vi "write_to_database.vi"(0 "heat_board_control in":refnum<class "heat_board_control.lvclass">, 5 "best setpoint":dbl, 7 "best manual laser":dbl, 11 "error in (no error)":errorcluster, 12 "database connection":path) -> (4 "heat_board_control out":refnum<class "heat_board_control.lvclass">, 15 "error out":errorcluster)   [LabVIEW 2015]
uses:
  heat_board_control.lvclass
  <vilib>/addons/database/Connection.llb/DB Tools Open Connec (Path).vi
  <vilib>/addons/database/NI_Database_API.lvlib
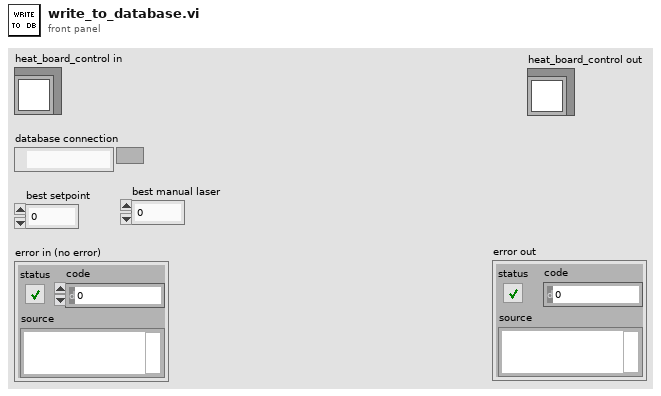
[diagram p1: front panel]
types:
  T1 = typedef "NI_Database_API.lvlib/Conn ObjectReference.ctl" = refnum<k1>
  T2 = cluster{"Rounded Number":dbl, "physical channel":refnum<k21>}
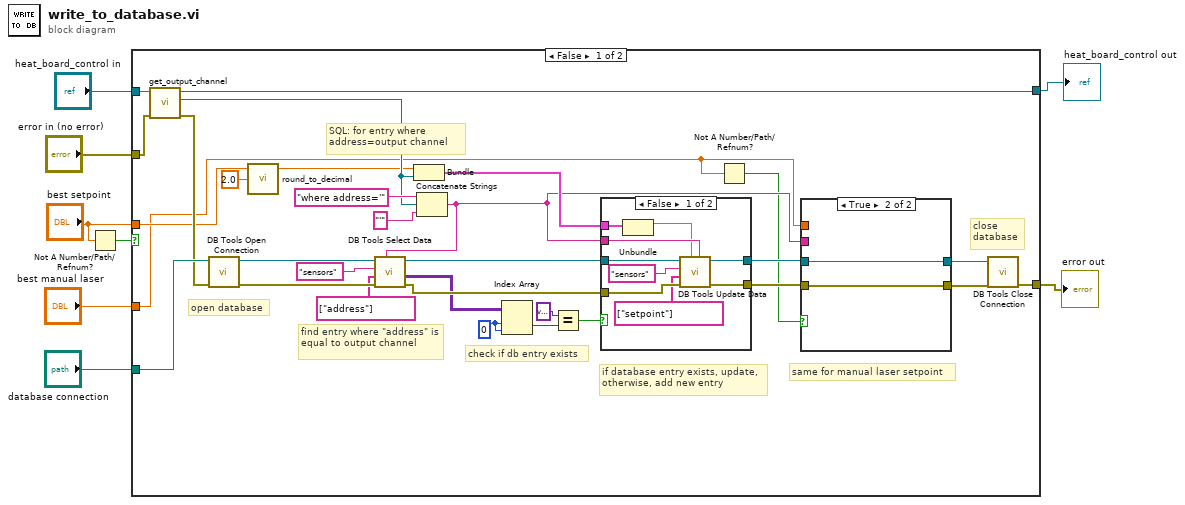
[diagram p0: block diagram]
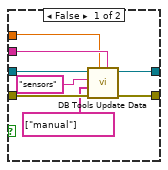
[diagram p2: hidden frame]
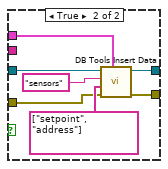
[diagram p3: hidden frame]
diagram:
  n1 = Not A Number/Path/Refnum?(number/path/refnum="best setpoint") -> (NaN/Path/Refnum?=w2:bool)
  n2 = case shown="False" w2 {
    tunnel: "error in (no error)" -> [w39 w66]
    tunnel: [w38 w66] -> w7
    tunnel: "heat_board_control in" -> [w37 w67]
    tunnel: "best setpoint" -> [w12 _]
    tunnel: "database connection" -> [w36 _]
    tunnel: [w21 w67] -> w5
    tunnel: "best manual laser" -> [w9 _]
    frame False {
      w24 = 0
      # "same for manual laser setpoint"
      # "close database"
      # "find entry where \"address\" is equal to output channel"
      # "open database"
      # "SQL: for entry where address=output channel"
      # "if database entry exists, update,\notherwise, add new entry"
      # "check if db entry exists"
      n3 = call-dynamic "get_output_channel.vi"("error in (no error)"=w39, "heat_board_control in"=w37) -> ("error out"=w34:errorcluster, "physical channel"=w25:refnum<k21>, "heat_board_control out"=w21:refnum<class "heat_board_control.lvclass">)  [unwired: 7 in]
      n4 = call-poly <vilib>:"DB Tools Open Connection.vi"("error in (no error)"=w34, "connection information"=w36) -> ("error out"=w30:errorcluster, "connection reference"=w33:T1)  [unwired: 6 in]
      n5 = call "round_to_decimal.vi"("Places after decimal point to round"=sgl 2.0, "Number to Round"=w12) -> ("Rounded Number"=w11:dbl)  [unwired: 3 in]
      n6 = Bundle("Rounded Number"=w11, "physical channel"=w25) -> (w35:T2)  [unwired: 1 in]
      n7 = Concatenate Strings("where address='" ("condition"), w25, "'") -> (w14:string)
      n8 = call <vilib>:"DB Tools Select Data.vi"("condition"=w14, "error in (no error)"=w30, "columns"=string[] ["address"], "table"="sensors", "connection reference"=w33) -> ("error out"=w29:errorcluster, "data"=w23:variant[][], "connection reference out"=w32:T1)  [unwired: 1 in]
      n9 = Index Array(array=w23, index (row)=w24, index (col)=w24) -> (element=w20:variant)
      n10 = Equal?(x=variant ("y"), y=w20) -> (x = y?=w22:bool)
      n11 = case shown="False" w22 {
        tunnel: w35 -> [w51 w65]
        tunnel: [w57 w63] -> w16
        tunnel: [w55 w62] -> w15
        tunnel: w32 -> [w58 w60]
        tunnel: w29 -> [w56 w59]
        tunnel: w14 -> [w52 _]
        frame False {
          n12 = Unbundle(w51) -> ("Rounded Number"=w50:dbl)  [unwired: 1 out]
          n13 = call <vilib>:"DB Tools Update Data.vi"("condition"=w52, "data"=w50, "error in (no error)"=w56, "columns"=string[] ["setpoint"], "table"="sensors", "connection reference"=w58) -> ("error out"=w55:errorcluster, "connection reference out"=w57:T1)  [unwired: 4 in]
        }
        frame True {
          n14 = call <vilib>:"DB Tools Insert Data.vi"("data"=w65, "error in (no error)"=w59, "columns"=string[] ["setpoint", "address"], "table"="sensors", "connection reference"=w60) -> ("error out"=w62:errorcluster, "connection reference out"=w63:T1)  [unwired: 5 in]
        }
      }
      n15 = Not A Number/Path/Refnum?(number/path/refnum=w9) -> (NaN/Path/Refnum?=w13:bool)
      n16 = case shown="True" w13 {
        tunnel: [w46 w49] -> w18
        tunnel: [w44 w48] -> w17
        tunnel: w16 -> [w47 w49]
        tunnel: w15 -> [w45 w48]
        tunnel: w14 -> [w41 _]
        tunnel: w9 -> [w40 _]
        frame False {
          n17 = call <vilib>:"DB Tools Update Data.vi"("condition"=w41, "data"=w40, "error in (no error)"=w45, "columns"=string[] ["manual"], "table"="sensors", "connection reference"=w47) -> ("error out"=w44:errorcluster, "connection reference out"=w46:T1)  [unwired: 4 in]
        }
        frame True {
        }
      }
      n18 = call <vilib>:"DB Tools Close Connection.vi"("error in (no error)"=w17, "connection reference"=w18) -> ("error out"=w38:errorcluster)  [unwired: 5 in]
    }
    frame True {
    }
  }
  "error out" <- w7
  "heat_board_control out" <- w5
